vi "校准条件设置.vi"() -> ()   [LabVIEW 2016, in "斯坦道总磷总氮.lvlib"]
uses:
  <vilib>/Utility/miscctls.llb/LVPointTypeDef.ctl
panel:
  in  "关闭":bool
  out "线性相关系数":dbl=0.999
  # "校准条件设置"
  # "说明：校准结果线性相关系数大于设定值，\n校准结果将自动写入仪器。"
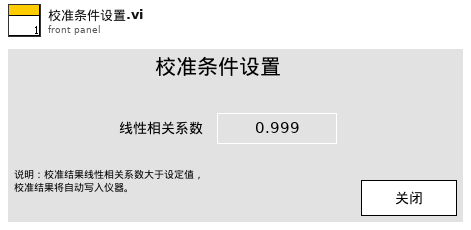
[diagram p1: front panel]
types:
  T1 = typedef "LVPointTypeDef.ctl" = cluster{"Horizontal":i16, "Vertical":i16}
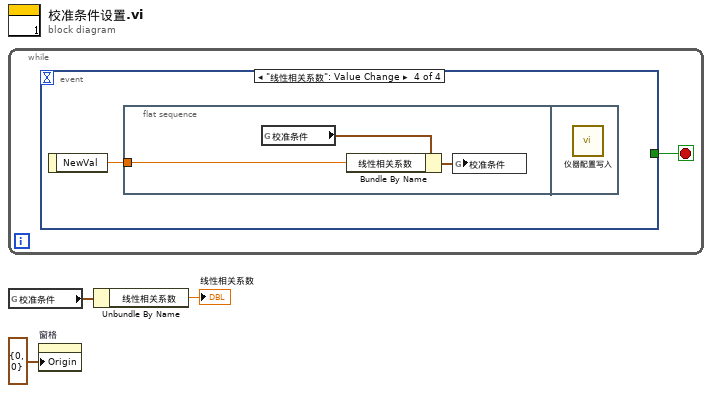
[diagram p0: block diagram]
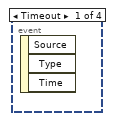
[diagram p2: hidden frame]
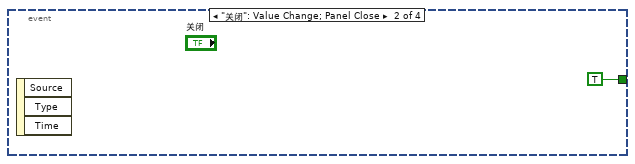
[diagram p3: hidden frame]
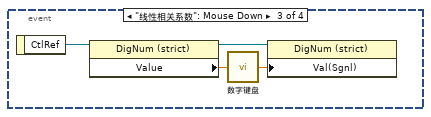
[diagram p4: hidden frame]
diagram:
  n1 = while {
    stop <- w4 stop-if-true
    n2 = event shown="[3] \"线性相关系数\": Value Change" {
      selector: _ -> [_ _ _ _]
      dyn-events: _ -> [_ _ _ _]
      timeout: _ -> [_ _ _ _]
      tunnel: [_ TRUE _ _] -> w4
      event Timeout {
        n3 = event-data() -> ()  [unwired: 1 in, 3 out]
      }
      event "关闭": Value Change; Panel Close {
        n4 = event-data() -> ()  [unwired: 1 in, 3 out]
      }
      event "线性相关系数": Mouse Down {
        n5 = event-data() -> ("CtlRef"=w9:refnum<vi>)  [unwired: 1 in]
        n6 = property class="DigNum (strict)"(reference=w9) -> (reference out=w7:refnum<vi>, "Value"=w8:dbl)  [unwired: 1 in, 1 out]
        n7 = call "数字键盘.vi"("OldNumber"=w8) -> ("NewNumber"=w6:dbl)
        n8 = property class="DigNum (strict)"(reference=w7, "Val(Sgnl)"=w6) -> ()  [unwired: 1 in, 2 out]
      }
      event "线性相关系数": Value Change {
        n9 = event-data() -> ("NewVal"=w10:dbl)  [unwired: 1 in]
        n10 = flat-sequence {
          tunnel: w10 -> [w11]
          frame #0 {
            n11 = global read "总磷总氮断电保存全局变量.vi" "校准条件"() -> (w13:cluster{"线性相关系数":dbl})
            n12 = Bundle By Name(cluster=w13, "线性相关系数"=w11) -> (w12:cluster{"线性相关系数":dbl})
            n13 = global write "总磷总氮断电保存全局变量.vi" "校准条件"(w12) -> ()
          }
          frame #1 {
            n14 = call "仪器配置写入.vi"() -> ()  [unwired: 11 in, 1 out]
          }
        }
      }
    }
  }
  n15 = global read "总磷总氮断电保存全局变量.vi" "校准条件"() -> (w3:cluster{"线性相关系数":dbl})
  n16 = property on="窗格" class="Pane"("Origin"=T1 {"Horizontal"=0, "Vertical"=0} ("原点")) -> ()  [unwired: 2 in, 2 out]
  n17 = Unbundle By Name(w3) -> ("线性相关系数"=→"线性相关系数":dbl)
